vi "Frequency (N Channels).vi"(8 "error in (no error)":errorcluster, 11 "waveforms":waveform(dbl)[](array[waveform])) -> (0 "error out":errorcluster, 3 "frequencies":dbl[](array[numeric]))   [LabVIEW 2013, in "NI_EP_Basic.lvlib"]
doc: "Calculates the fundamental frequency of a voltage or current signal. Wire data to the <B>waveform</B> input to determine the polymorphic instance to use or manually select the instance."
uses:
  <vilib>/addons/Electrical Power/Basic/NI_EP_Basic.lvlib
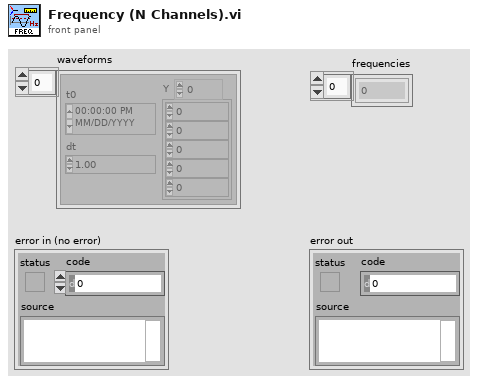
[diagram p1: front panel]
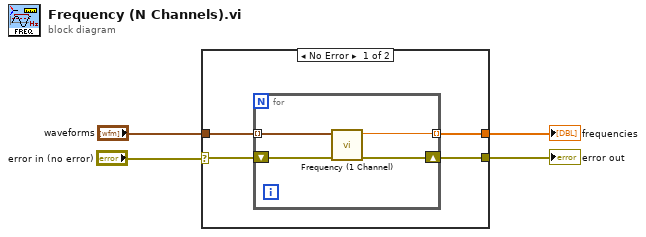
[diagram p0: block diagram]
diagram:
  n1 = case shown="No Error" "error in (no error)" {
    selector: "error in (no error)" -> [w7 w13]
    tunnel: "waveforms" -> [w8 _]
    tunnel: [w6 _] -> w2
    tunnel: [w5 w13] -> w1
    frame No Error {
      n2 = for {
        tunnel: w8 -> [w12] mode=indexing
        shift-right: [w10] -> w5
        shift-left: w7 -> [w11]
        tunnel: [w9] -> w6 mode=indexing
        n3 = call <vilib>:"Frequency (1 Channel).vi"("error in (no error)"=w11, "waveform"=w12) -> ("error out"=w10:errorcluster, "frequency"=w9:dbl)  [unwired: 8 in]
      }
    }
    frame Error {
    }
  }
  "frequencies" <- w2
  "error out" <- w1
